vi "Insert Subscriber by Name.vi"(8 "error in (no error)":errorcluster, 9 "Subscriber":refnum<class "Message Transport Interface.lvclass">, 10 "Topic Name":string, 11 "Subscriber Index Look Up Table in":refnum<class "Subscriber Look Up Table.lvclass">) -> (0 "error out":errorcluster, 2 "Replaced?":bool, 3 "Subscriber Index Look Up Table out":refnum<class "Subscriber Look Up Table.lvclass">)   [LabVIEW 2016, in "Stream Mediator.lvlib" / "Subscriber Look Up Table.lvclass"]
doc: "--\nCopyright © 2017 Composed SystemsI All rights reserved.\n\nAuthor: Jon McBee <jon.mcbee@composed.io>\n\nThis library is provided \"AS IS\" ,WITHOUT WARRANTIES OR\nCONDITIONS OF ANY KIND, either express or implied.\n\nComposed Systems -- composed.io\n\nStream 0.0.1.1\nJon McBee - Composed Systems\nCopyright (c) 2017, Composed Systems"
uses:
  <userlib>/Composed Systems/Stream/Mediator/Classes/Subscriber Look Up Table/Subscriber Look Up Table.lvclass
  C:/Program Files (x86)/National Instruments/LabVIEW 2016/user.lib/Composed Systems/Stream/Look Up Table/Look Up Table/Look Up Table.lvclass
  <userlib>/Composed Systems/Stream/Mediator/Classes/Message Transport Interface/Message Transport Interface.lvclass
  <userlib>/Composed Systems/Stream/Look Up Table/Look Up Table/Look Up Table.lvclass
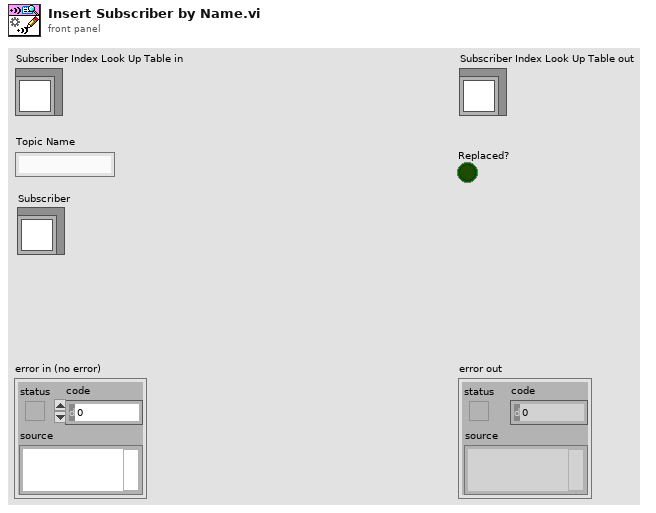
[diagram p1: front panel]
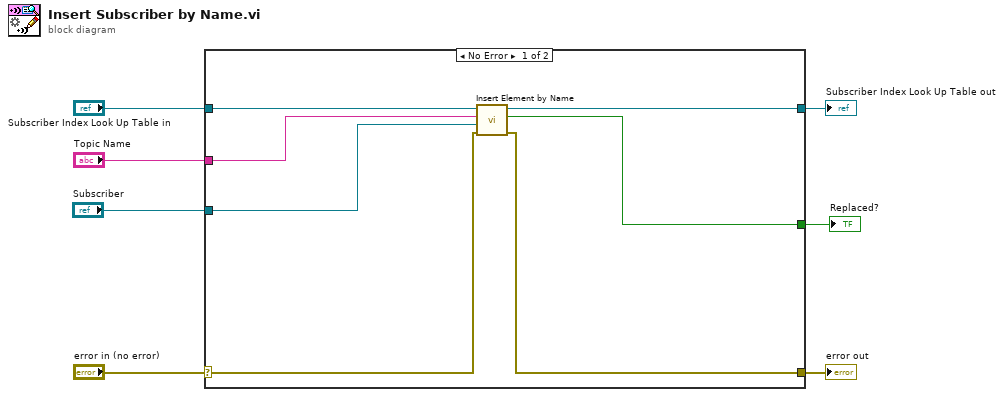
[diagram p0: block diagram]
diagram:
  n1 = case shown="No Error" "error in (no error)" {
    selector: "error in (no error)" -> [w12 w16]
    tunnel: [w11 w16] -> w6
    tunnel: [w13 w15] -> w4
    tunnel: "Subscriber Index Look Up Table in" -> [w14 w15]
    tunnel: "Topic Name" -> [w9 _]
    tunnel: "Subscriber" -> [w8 _]
    tunnel: [w10 _] -> w2
    frame No Error {
      n2 = call <userlib>:"Insert Element by Name.vi"("error in (no error)"=w12, "Variant"=w8, "Name"=w9, "Look Up Table in"=w14) -> ("error out"=w11:errorcluster, "Replaced?"=w10:bool, "Look Up Table out"=w13:refnum<class "Subscriber Look Up Table.lvclass">)  [unwired: 5 in]
    }
    frame Error {
    }
  }
  "error out" <- w6
  "Subscriber Index Look Up Table out" <- w4
  "Replaced?" <- w2
